vi "TW Update Library Names.vi"(6 "Libraries":T1(array[cluster]), 8 "error in":errorcluster, 9 "Replace Subname":string="Template", 10 "New Subname":string, 11 "Library Map":map{string, refnum<vi>}(c390)) -> (0 "error out":errorcluster, 3 "Library Map":map{string, refnum<vi>}(c390))   [LabVIEW 2021, in "Plugin Generator.lvlib"]
uses:
  Plugin Generator.lvlib
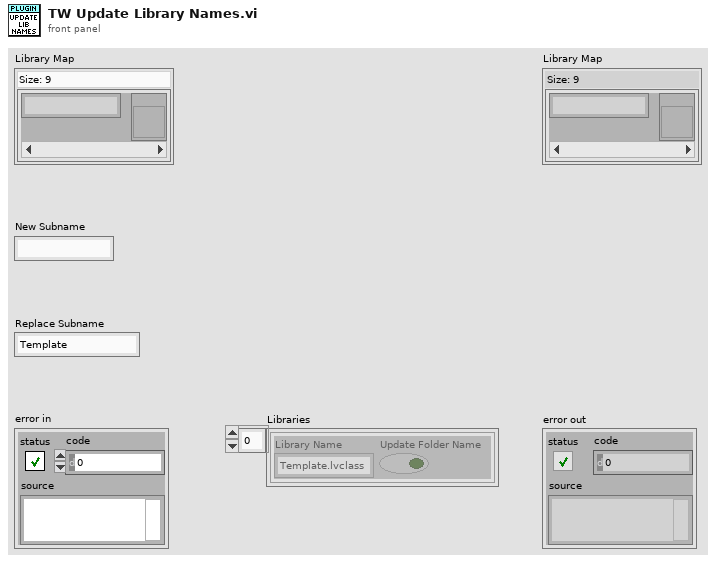
[diagram p1: front panel]
types:
  T1 = cluster{"Library Name":string, "Update Folder Name":bool}[]
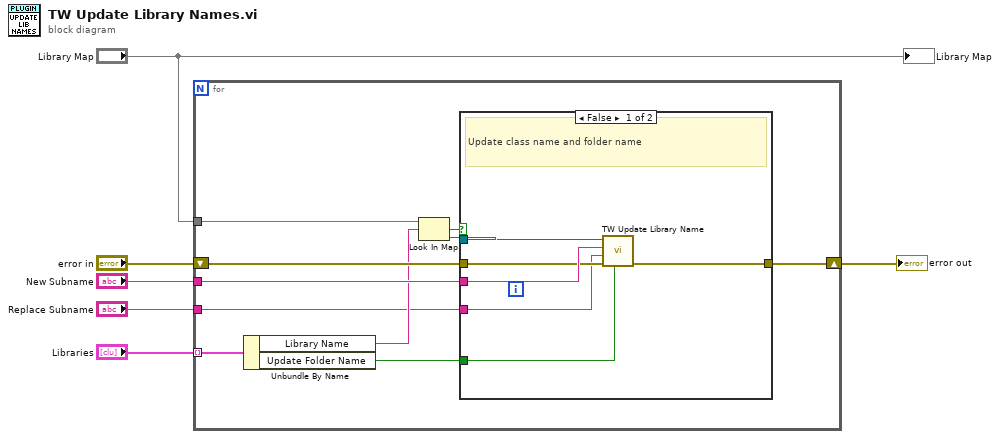
[diagram p0: block diagram]
diagram:
  n1 = for {
    tunnel: "Libraries" -> [w10] mode=indexing
    tunnel: "Library Map" -> [w16]
    tunnel: "New Subname" -> [w12]
    shift-right: [w14] -> w2
    shift-left: "error in" -> [w11]
    tunnel: "Replace Subname" -> [w7]
    n2 = Unbundle By Name(w10) -> ("Library Name"=w9:string, "Update Folder Name"=w8:bool)
    n3 = Look In Map(map=w16, key=w9) -> (key not found?=w15:bool, value=w13:refnum<vi>)  [unwired: 1 in]
    n4 = case shown="False" w15 {
      tunnel: [w22 w23] -> w14
      tunnel: w13 -> [w21 _]
      tunnel: w12 -> [w20 _]
      tunnel: w11 -> [w19 w23]
      tunnel: w8 -> [w18 _]
      tunnel: w7 -> [w17 _]
      frame False {
        # "Update class name and folder name"
        n5 = call "TW Update Library Name.vi"("Update Folder Name"=w18, "error in (no error)"=w19, "Replace Subname"=w17, "New Subname"=w20, "Library in"=w21) -> ("error out"=w22:errorcluster)  [unwired: 6 in]
      }
      frame True {
        # "Could add error here since expected folder was not found"
      }
    }
  }
  "error out" <- w2
  "Library Map" <- "Library Map"
